vi "Push Explode Left.vi"(8 "error in (no error)":errorcluster, 10 "Explode Result In":T1, 11 "SnailNum in":refnum<class "SnailNum.lvclass">) -> (0 "error out":errorcluster, 2 "Explode Result":T1, 3 "SnailNum out":refnum<class "SnailNum.lvclass">)   [LabVIEW 2020, in "SnailNum.lvclass"]
uses:
  SnailNum.lvclass
  Explode Result.ctl
  SnailNum.lvclass/SnailNum.ctl
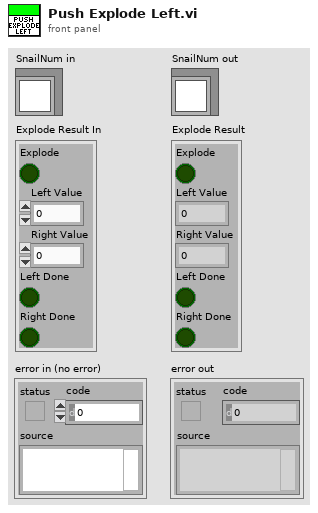
[diagram p1: front panel]
types:
  T1 = typedef "SnailNum.lvclass/Explode Result.ctl" = cluster{"Explode":bool, "Left Value":i64, "Right Value":i64, "Left Done":bool, "Right Done":bool}
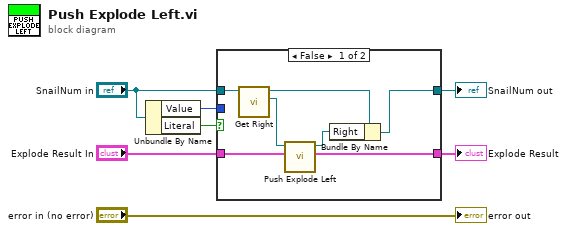
[diagram p0: block diagram]
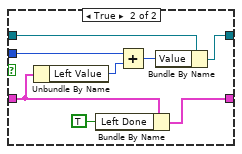
[diagram p2: hidden frame]
diagram:
  n1 = Unbundle By Name("SnailNum in") -> ("Value"=w6:i64, "Literal"=w5:bool)
  n2 = case shown="False" w5 {
    tunnel: w6 -> [_ w19]
    tunnel: "SnailNum in" -> [w14 w16]
    tunnel: "Explode Result In" -> [w12 w22]
    tunnel: [w11 w20] -> w1
    tunnel: [w9 w15] -> w2
    frame False {
      n3 = call "Get Right.vi"("SnailNum in"=w14) -> ("Right"=w13:refnum<class "SnailNum.lvclass">, "SnailNum out"=w10:refnum<class "SnailNum.lvclass">)  [unwired: 8 in, 1 out]
      n4 = call "Push Explode Left.vi"("Explode Result In"=w12, "SnailNum in"=w13) -> ("Explode Result"=w11:T1, "SnailNum out"=w8:refnum<class "SnailNum.lvclass">)  [unwired: 7 in, 1 out]
      n5 = Bundle By Name(cluster=w10, "Right"=w8) -> (w9:refnum<class "SnailNum.lvclass">)
    }
    frame True {
      n6 = Unbundle By Name(w22) -> ("Left Value"=w18:i64)
      n7 = Bundle By Name(cluster=w22, "Left Done"=TRUE) -> (w20:T1)
      n8 = Add(x=w19, y=w18) -> (x+y=w17:i64)
      n9 = Bundle By Name(cluster=w16, "Value"=w17) -> (w15:refnum<class "SnailNum.lvclass">)
    }
  }
  "SnailNum out" <- w2
  "Explode Result" <- w1
  "error out" <- "error in (no error)"
